vi "Fpga-AXI-Stream-Test.old.vi"() -> ()   [LabVIEW 2017]
uses:
  <vilib>/Platform/TimedLoop/XDataNode/timing_clust.ctl
  <vilib>/Platform/TimedLoop/XDataNode/nitl_modes.ctl
  <vilib>/Platform/TimedLoop/XDataNode/wakeup.ctl
  <vilib>/rvi/IPIntegrationNode/IPINode_Typedef/niFpgaIPINodeSupportedFamilies.ctl
  <vilib>/rvi/Emulation/niFpgaSctlEmulationGetInTimedLoop.vi
  <vilib>/rvi/Emulation/niFpgaEmulationReportErrorSimple.vi
  <vilib>/rvi/Emulation/niFpgaGetClockAttributes.vi
  <vilib>/rvi/Emulation/niFpgaCriticalErrorInLSC.vi
  <vilib>/rvi/IPIntegrationNode/IPINode_Utilities/niFpgaIPINodeSimCore.vi
  <vilib>/Platform/TimedLoop/XDataNode/XDataNode.xnode
  <vilib>/rvi/IPIntegrationNode/IPINode_Xnode/niFpgaIPINode.xnode
  IP_BlockSimFiles/xsim.dir/d_microblaze_wrapper_top/xsimkFD8EF92288A74FC0A132AE6276DBDF30.dll
  <vilib>/Platform/TimedLoop/XDataNode/XDNodeRunTimeDep.lvlib
panel:
  in  "AXI_STR_RXD_tlast":bool
  in  "AXI_STR_RXD_tdata":u32
  in  "AXI_STR_RXD_tvalid":bool
  in  "AXI_STR_TXD_tready":bool
  out "TXD_tvalid":u16
  out "TXD_tlast":u16
  out "TXD_tdata":u32
  out "RXD_tready":u16
  out "ACLK":u16
  in  "gpio1_tri_i":u32
  out "gpio2_tri_o":u32
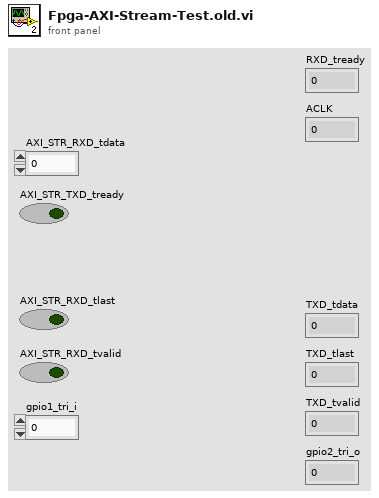
[diagram p1: front panel]
types:
  T1 = typedef "XDNodeRunTimeDep.lvlib/timing_clust.ctl" = cluster{"Expected End [f-1]":u64, "Actual End [f-1]":u64, "Finished Late? [f-1]":bool, "Expected End [i-1]":u64, "Actual End [i-1]":u64, "Finished Late? [i-1]":bool, "Expected Start [i]":u64, "Actual Start [i]":u64, "Expected Start [f]":u64, "Actual Start [f]":u64, "Source Name":string, "Structure Name":string, "Period":i64, "Deadline":i64, "Offset":i64, "Start":i64, "Priority":i32, "Timeout":i32, "Mode":T2, "Wakeup Reason":T3, "Error":errorcluster, "Source Type":string, "Secondary Source Type":string, "Global End Time":u64, "Global Start Time":u64, "Frame Duration":u64, "Iteration Duration":u64, "Assigned CPU":i32, "I/O Scan Engine Mode":u32}
  T2 = typedef "XDNodeRunTimeDep.lvlib/nitl_modes.ctl" = enum32{"No Change", "Process missed periods, maintain original phase", "Discard missed periods, maintain original phase", "Process missed periods, ignore original phase", "Discard missed periods, ignore original phase"}
  T3 = typedef "XDNodeRunTimeDep.lvlib/wakeup.ctl" = enum32{"Normal", "Aborted", "Asynchronous wakeup", "Timing source error", "Timed loop error", "Timeout"}
  T4 = typedef "niFpgaIPINodeSupportedFamilies.ctl" = cluster{"unlimited?":bool, "supported targets":string[]}
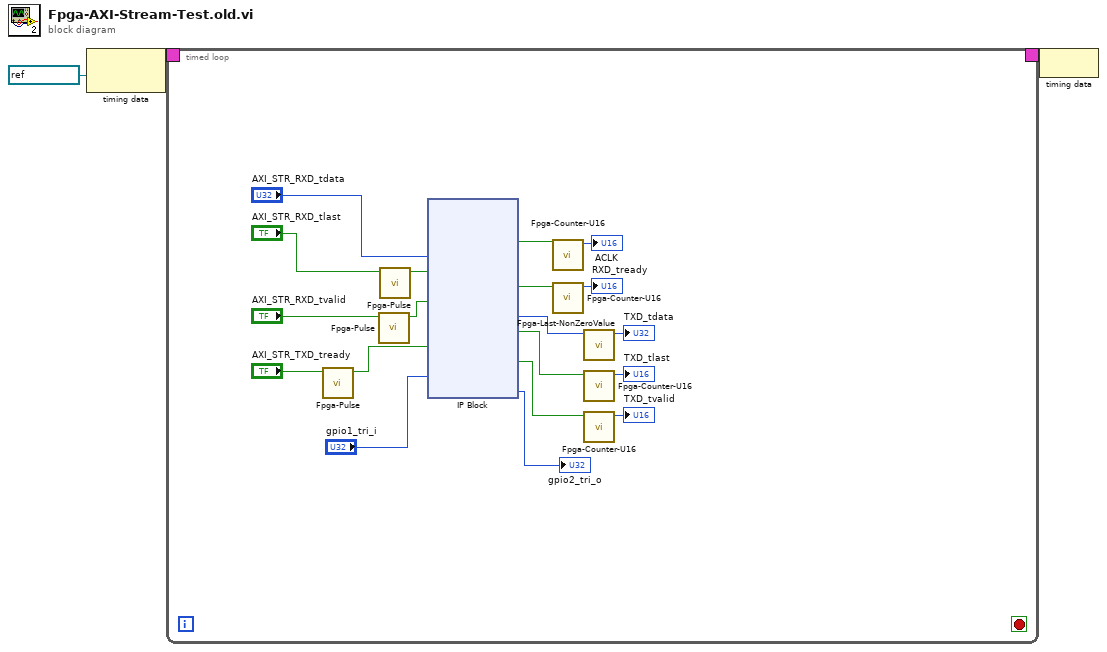
[diagram p0: block diagram]
diagram:
  n1 = node-c288(refnum<k21> "100MHz" ("Source Name")) -> (w3:T1)
  n2 = timed-loop {
    timing: w3 -> [_]
    timing-out: [_] -> w2
    stop <- _ stop-if-true
    n3 = call "Fpga-Pulse.vi"("AXI_STR_TXD_tready"="AXI_STR_TXD_tready") -> ("Boolean"=w8:bool)  [unwired: 10 in]
    n4 = call "Fpga-Pulse.vi"("AXI_STR_TXD_tready"="AXI_STR_RXD_tvalid") -> ("Boolean"=w7:bool)  [unwired: 10 in]
    n5 = call "Fpga-Pulse.vi"("AXI_STR_TXD_tready"="AXI_STR_RXD_tlast") -> ("Boolean"=w5:bool)  [unwired: 10 in]
    n6 = xnode ("IP Block")("AXI_STR_RXD_tdata"="AXI_STR_RXD_tdata", "AXI_STR_RXD_tlast"=w5, "AXI_STR_RXD_tvalid"=w7, "AXI_STR_TXD_tready"=w8, "gpio1_tri_i"="gpio1_tri_i") -> ("ACLK"=w20:bool, "AXI_STR_RXD_tready"=w19:bool, "AXI_STR_TXD_tdata"=w16:u32, "AXI_STR_TXD_tlast"=w18:bool, "AXI_STR_TXD_tvalid"=w17:bool, "gpio2_tri_o"=→"gpio2_tri_o":u32)  [unwired: 1 in]
    n7 = call "Fpga-Counter-U16.vi"("d_mcs_i\\IO_BUS_read_strobe"=w20) -> ("Numeric"=→"ACLK":u16)  [unwired: 10 in]
    n8 = call "Fpga-Counter-U16.vi"("d_mcs_i\\IO_BUS_read_strobe"=w19) -> ("Numeric"=→"RXD_tready":u16)  [unwired: 10 in]
    n9 = call "Fpga-Last-NonZeroValue.vi"("d_mcs_i\\IO_BUS_write_data in"=w16) -> ("d_mcs_i\\IO_BUS_write_data out"=→"TXD_tdata":u32)  [unwired: 10 in]
    n10 = call "Fpga-Counter-U16.vi"("d_mcs_i\\IO_BUS_read_strobe"=w18) -> ("Numeric"=→"TXD_tlast":u16)  [unwired: 10 in]
    n11 = call "Fpga-Counter-U16.vi"("d_mcs_i\\IO_BUS_read_strobe"=w17) -> ("Numeric"=→"TXD_tvalid":u16)  [unwired: 10 in]
  }
  n12 = node-c288(w2) -> ()
